vi "Check Currency Limit.vi"(8 "error in (no error)":errorcluster, 10 "Enum":T1, 11 "Balance":dbl) -> (0 "error out":errorcluster, 2 "Max Exceeded?":bool, 3 "New Balance":dbl)   [LabVIEW 2026]
uses:
  controls/Currency Enum.ctl
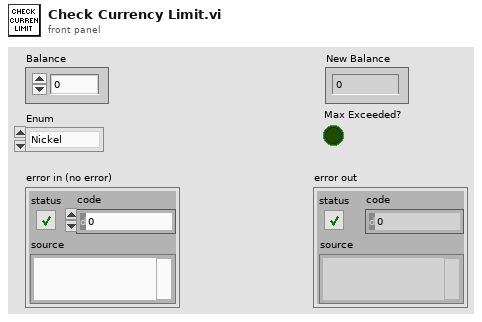
[diagram p1: front panel]
types:
  T1 = typedef "Currency Enum.ctl" = enum16{"Nickel", "Dime", "Quarter", "Dollar"}
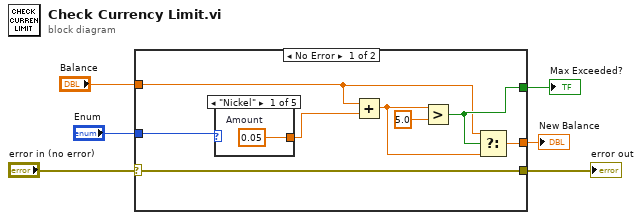
[diagram p0: block diagram]
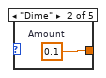
[diagram p2: hidden frame]
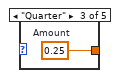
[diagram p3: hidden frame]
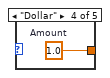
[diagram p4: hidden frame]
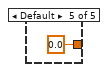
[diagram p5: hidden frame]
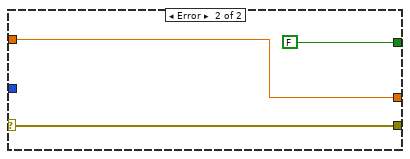
[diagram p6: hidden frame]
diagram:
  n1 = case shown="No Error" "error in (no error)" {
    selector: "error in (no error)" -> [w14 w22]
    tunnel: [w14 w22] -> w5
    tunnel: "Balance" -> [w11 w20]
    tunnel: [w12 FALSE] -> w3
    tunnel: [w9 w20] -> w2
    tunnel: "Enum" -> [w8 _]
    frame No Error {
      n2 = case shown="\"Nickel\"" w8 {
        tunnel: [w15 w16 w17 w18 0.0 ("Amount")] -> w7
        frame "Nickel" {
          w15 = 0.05  # Amount
        }
        frame "Dime" {
          w16 = 0.1  # Amount
        }
        frame "Quarter" {
          w17 = 0.25  # Amount
        }
        frame "Dollar" {
          w18 = 1.0  # Amount
        }
        frame Default {
        }
      }
      n3 = Add(x=w11, y=w7) -> (x+y=w10:dbl)
      n4 = Greater?(x=w10, y=5.0) -> (0:w12:bool)
      n5 = Select(t=w11, s=w12, f=w10) -> (s? t:f=w9:dbl)
    }
    frame Error {
    }
  }
  "error out" <- w5
  "Max Exceeded?" <- w3
  "New Balance" <- w2
